vi "Get Log Directory Path.vi"(8 "error in (no error)":errorcluster, 11 "session in":refnum<class "Plugin Session.lvclass">) -> (0 "error out":errorcluster, 2 "Log file directory path":path, 3 "session out":refnum<class "Plugin Session.lvclass">)   [LabVIEW 2021, in "Game of Life.lvlib"]
doc: "Gets the directory path for log file"
uses:
  Game of Life.lvlib
  <vilib>/Plug-In SDKs/InstrumentStudio/Plugin Session.lvclass
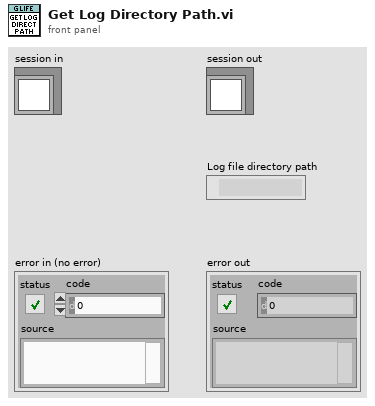
[diagram p1: front panel]
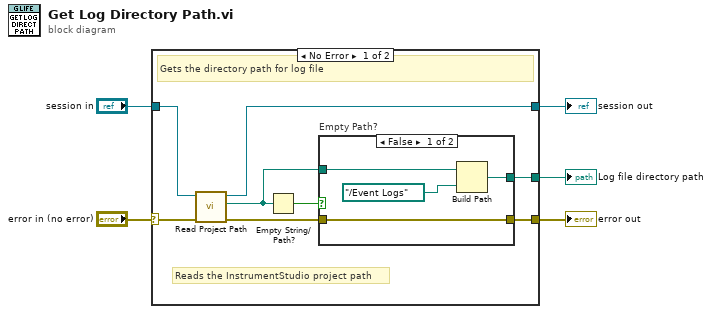
[diagram p0: block diagram]
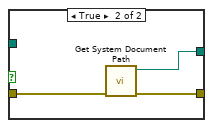
[diagram p2: hidden frame]
diagram:
  n1 = case shown="No Error" "error in (no error)" {
    selector: "error in (no error)" -> [w12 w21]
    tunnel: [w13 w21] -> w5
    tunnel: "session in" -> [w10 w20]
    tunnel: [w9 w20] -> w2
    tunnel: [w6 _] -> w1
    frame No Error {
      # "Reads the InstrumentStudio project path"
      # "Gets the directory path for log file"
      n2 = call <vilib>:"Read Project Path.vi"("error in (no error)"=w12, "Session in"=w10) -> ("error out"=w11:errorcluster, "Project Path"=w7:path, "Session out"=w9:refnum<class "Plugin Session.lvclass">)  [unwired: 7 in]
      n3 = Empty String/Path?(string/path=w7) -> (empty?=w8:bool)
      n4 = case "Empty Path?" shown="False" w8 {
        tunnel: w11 -> [w17 w19]
        tunnel: [w17 w19] -> w13
        tunnel: w7 -> [w16 _]
        tunnel: [w14 w18] -> w6
        frame False {
          n5 = Build Path(base path=w16, name or relative path=path "../Event Logs") -> (appended path=w14:path)
        }
        frame True {
          n6 = call "Get System Document Path.vi"() -> ("Public Path"=w18:path)  [unwired: 11 in]
        }
      }
    }
    frame Error {
    }
  }
  "error out" <- w5
  "Log file directory path" <- w1
  "session out" <- w2
